vi "test-Vision-Utils-Test3.vi"() -> (3 "All Passed":bool)   [LabVIEW 2019]
uses:
  <vilib>/Rock Robotics/WPI/ThirdParty/JAS_Junk/TrajLib/VI/Translation3d_Create_Default.vi
  <vilib>/Rock Robotics/WPI/ThirdParty/JAS_Junk/TrajLib/VI/Rotation3d_Create_Default.vi
  <vilib>/Rock Robotics/WPI/ThirdParty/JAS_Junk/TrajLib/VI/Pose3d_New_Trans3dRot3d.vi
  <vilib>/Rock Robotics/WPI/ThirdParty/JAS_Junk/TrajLib/Rotation2d_CreateAngle.vi
  <vilib>/Rock Robotics/WPI/ThirdParty/JAS_Junk/TrajLib/VI/Quaternion_New.vi
  <vilib>/Rock Robotics/WPI/ThirdParty/JAS_Junk/TrajLib/VI/Quaternion_Get_All.vi
  <vilib>/Rock Robotics/WPI/ThirdParty/JAS_Junk/TrajLib/VI/Rotation3d_GetQuaterion.vi
  <vilib>/Rock Robotics/WPI/ThirdParty/JAS_Junk/TrajLib/VI/Pose3d_getTranslation3d.vi
  <vilib>/Rock Robotics/WPI/ThirdParty/JAS_Junk/TrajLib/VI/Translation3d_GetXYZ.vi
  <vilib>/Rock Robotics/WPI/ThirdParty/JAS_Junk/TrajLib/VI/Translation3d_RotateBy.vi
  <vilib>/Rock Robotics/WPI/ThirdParty/JAS_Junk/TrajLib/VI/Rotation3d_Minus.vi
  <vilib>/Rock Robotics/WPI/ThirdParty/JAS_Junk/TrajLib/VI/CompVisionUtil_EstimateFieldToCamera.vi
  <vilib>/Rock Robotics/WPI/ThirdParty/JAS_Junk/TrajLib/VI/Pose3d_TransformBy.vi
  <vilib>/Rock Robotics/WPI/ThirdParty/JAS_Junk/TrajLib/Rotation2d_GetAngleCosSin.vi
  <vilib>/Rock Robotics/WPI/ThirdParty/JAS_Junk/TrajLib/VI/Quaternion_New_Default.vi
  <vilib>/Rock Robotics/WPI/ThirdParty/JAS_Junk/TrajLib/VI/Quaternion_Times.vi
  <vilib>/Rock Robotics/WPI/ThirdParty/JAS_Junk/TrajLib/VI/Quaternion_Inverse.vi
  <vilib>/Rock Robotics/WPI/ThirdParty/JAS_Junk/TrajLib/VI/Rotation3d_UnaryMinus.vi
  <vilib>/Rock Robotics/WPI/ThirdParty/JAS_Junk/TrajLib/VI/Rotation3d_RotateBy.vi
  <vilib>/Rock Robotics/WPI/ThirdParty/JAS_Junk/TrajLib/VI/Transform3d_Inverse.vi
  <vilib>/Rock Robotics/WPI/ThirdParty/JAS_Junk/TrajLib/VI/Transform3d_GetTranslation3d.vi
  <vilib>/Rock Robotics/WPI/ThirdParty/JAS_Junk/TrajLib/VI/Transform3d_GetRotation3d.vi
  <vilib>/Rock Robotics/WPI/ThirdParty/JAS_Junk/TrajLib/VI/Translation3d_Plus.vi
  <vilib>/Rock Robotics/WPI/ThirdParty/JAS_Junk/TrajLib/VI/Rotation3d_Plus.vi
  <vilib>/Rock Robotics/WPI/ThirdParty/JAS_Junk/TrajLib/VI/Rotation3d_Create_Quaternion.vi
  <vilib>/Rock Robotics/WPI/ThirdParty/JAS_Junk/TrajLib/VI/Translation3d_UnaryMinus.vi
  <vilib>/Rock Robotics/WPI/ThirdParty/JAS_Junk/TrajLib/VI/Quaternion_Normalize.vi
  <vilib>/Rock Robotics/WPI/ThirdParty/JAS_Junk/TrajLib/Trajectory_Library.lvlib
panel:
  out "Test 1":bool
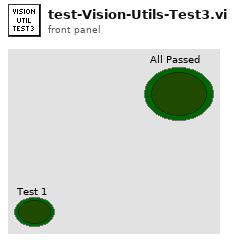
[diagram p1: front panel]
types:
  T1 = typedef "Trajectory_Library.lvlib/ROTATION3D.ctl" = cluster{"Q_quaternion":T2}
  T2 = typedef "Trajectory_Library.lvlib/QUATERNION.ctl" = cluster{"R":dbl, "V":dbl[]}
  T3 = typedef "Trajectory_Library.lvlib/POSE3D.ctl" = cluster{"Translation3d":T4, "Rotation3d":T1}
  T4 = typedef "Trajectory_Library.lvlib/TRANSLATION3D.ctl" = cluster{"X":dbl, "Y":dbl, "Z":dbl}
  T5 = typedef "Trajectory_Library.lvlib/TRANSFORM3D.ctl" = cluster{"TRANSLATION3D":T4, "ROTATION3D":T1, "XF":bool}
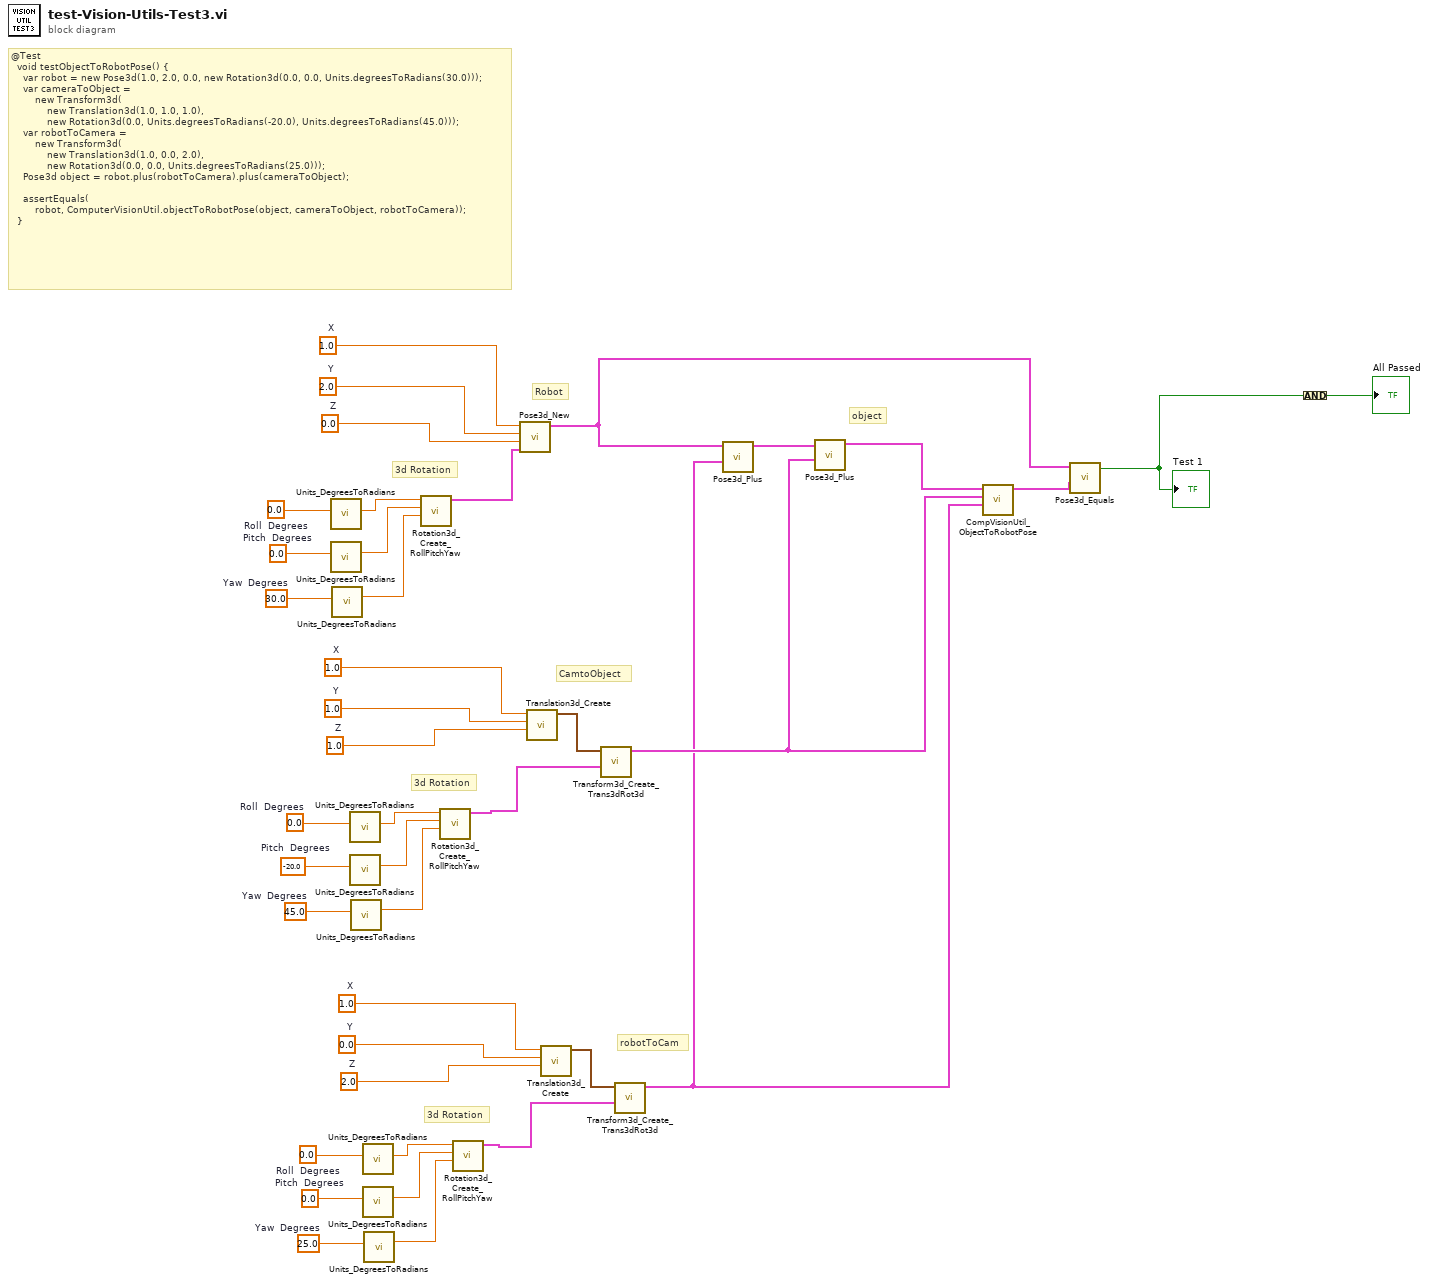
[diagram p0: block diagram]
diagram:
  w10 = 0.0  # Roll  Degrees
  w11 = 0.0  # Pitch  Degrees
  w12 = 25.0  # Yaw  Degrees
  w16 = 0.0  # Roll  Degrees
  w17 = -20.0  # Pitch  Degrees
  w18 = 45.0  # Yaw  Degrees
  w23 = 0.0  # Roll  Degrees
  w24 = 0.0  # Pitch  Degrees
  w25 = 30.0  # Yaw  Degrees
  w32 = 1.0  # X
  w31 = 0.0  # Y
  w30 = 2.0  # Z
  w36 = 1.0  # X
  w35 = 1.0  # Y
  w34 = 1.0  # Z
  w39 = 1.0  # X
  w38 = 2.0  # Y
  w37 = 0.0  # Z
  # "object"
  # "robotToCam"
  # "CamtoObject"
  # "3d Rotation"
  # "3d Rotation"
  # "3d Rotation"
  # "Robot"
  # "@Test\n  void testObjectToRobotPose() {\n    var robot = new Pose3d(1.0, 2.0, 0.0, new Rotation3d(0.0, 0.0, Units.degreesToRadians(30.0)));\n    var cameraToObject =\n        new Transform3d(\n            new Translation3d(1.0, 1.0, 1.0),\n            new Rotation3d(0.0, Units.degreesToRadians(-20.0), Units.degreesToRadians(45.0)));\n    var robotToCamera =\n        new Transform3d(\n            new Translation3d(1.0, 0.0, 2.0),\n            new Rotation3d(0.0, 0.0, Units.degreesToRadians(25.0)));\n    Pose3d object = robot.plus(robotToCamera).plus(cameraToObject);\n\n    assertEquals(\n        robot, ComputerVisionUtil.objectToRobotPose(object, cameraToObject, robotToCamera));\n  }"
  n1 = call <vilib>:"Units_DegreesToRadians.vi"("Degrees"=w23) -> ("Radians"=w26:dbl)  [unwired: 10 in]
  n2 = call <vilib>:"Units_DegreesToRadians.vi"("Degrees"=w24) -> ("Radians"=w27:dbl)  [unwired: 10 in]
  n3 = call <vilib>:"Units_DegreesToRadians.vi"("Degrees"=w25) -> ("Radians"=w28:dbl)  [unwired: 10 in]
  n4 = call <vilib>:"Units_DegreesToRadians.vi"("Degrees"=w16) -> ("Radians"=w19:dbl)  [unwired: 10 in]
  n5 = call <vilib>:"Units_DegreesToRadians.vi"("Degrees"=w17) -> ("Radians"=w20:dbl)  [unwired: 10 in]
  n6 = call <vilib>:"Units_DegreesToRadians.vi"("Degrees"=w18) -> ("Radians"=w21:dbl)  [unwired: 10 in]
  n7 = call <vilib>:"Units_DegreesToRadians.vi"("Degrees"=w10) -> ("Radians"=w13:dbl)  [unwired: 10 in]
  n8 = call <vilib>:"Units_DegreesToRadians.vi"("Degrees"=w11) -> ("Radians"=w14:dbl)  [unwired: 10 in]
  n9 = call <vilib>:"Units_DegreesToRadians.vi"("Degrees"=w12) -> ("Radians"=w15:dbl)  [unwired: 10 in]
  n10 = call <vilib>:"Rotation3d_Create_RollPitchYaw.vi"("Yaw"=w28, "Pitch"=w27, "Roll"=w26) -> ("Rotation3d"=w22:T1)  [unwired: 8 in]
  n11 = call <vilib>:"Rotation3d_Create_RollPitchYaw.vi"("Yaw"=w21, "Pitch"=w20, "Roll"=w19) -> ("Rotation3d"=w8:T1)  [unwired: 8 in]
  n12 = call <vilib>:"Rotation3d_Create_RollPitchYaw.vi"("Yaw"=w15, "Pitch"=w14, "Roll"=w13) -> ("Rotation3d"=w9:T1)  [unwired: 8 in]
  n13 = call <vilib>:"Pose3d_New.vi"("Rotation3d"=w22, "z"=w37, "Y"=w38, "X"=w39) -> ("out Pose3d"=w2:T3)  [unwired: 7 in]
  n14 = call <vilib>:"Translation3d_Create.vi"("Z"=w34, "Y"=w35, "X"=w36) -> ("TRANSLATION3D"=w33:T4)  [unwired: 8 in]
  n15 = call <vilib>:"Translation3d_Create.vi"("Z"=w30, "Y"=w31, "X"=w32) -> ("TRANSLATION3D"=w29:T4)  [unwired: 8 in]
  n16 = call <vilib>:"Transform3d_Create_Trans3dRot3d.vi"("Rotation3d"=w8, "Translation3d"=w33) -> ("Transform3d"=w5:T5)  [unwired: 9 in]
  n17 = call <vilib>:"Transform3d_Create_Trans3dRot3d.vi"("Rotation3d"=w9, "Translation3d"=w29) -> ("Transform3d"=w4:T5)  [unwired: 9 in]
  n18 = call <vilib>:"Pose3d_Plus.vi"("other Transform3d"=w4, "in Pose3d"=w2) -> ("out Pose3d"=w7:T3)  [unwired: 9 in]
  n19 = call <vilib>:"Pose3d_Plus.vi"("other Transform3d"=w5, "in Pose3d"=w7) -> ("out Pose3d"=w6:T3)  [unwired: 9 in]
  n20 = call <vilib>:"CompVisionUtil_ObjectToRobotPose.vi"("RobotToCamera"=w4, "CameraToObject"=w5, "ObjectInField"=w6) -> ("ObjectToRobotPose"=w3:T3)  [unwired: 8 in]
  n21 = call <vilib>:"Pose3d_Equals.vi"("other Pose3d"=w3, "in Pose3d"=w2) -> ("Equals"=w1:bool)  [unwired: 9 in]
  "Test 1" <- w1
  n22 = Compound Arithmetic op=AND(w1) -> (→"All Passed":bool)
